vi "_emi_GFV Loop Running.vi"(0 "Loop Index/Numb":u16, 1 "Action(Get Index)":T1=enum."Get index", 7 "Loop Running In(F)":bool, 11 "error in (no error)":errorcluster) -> (4 "Index out":u16, 8 "Loop Running Out":bool, 10 "Size":i32, 15 "error out":errorcluster)   [LabVIEW 2011]
uses:
  _emi_Loop control int action.ctl
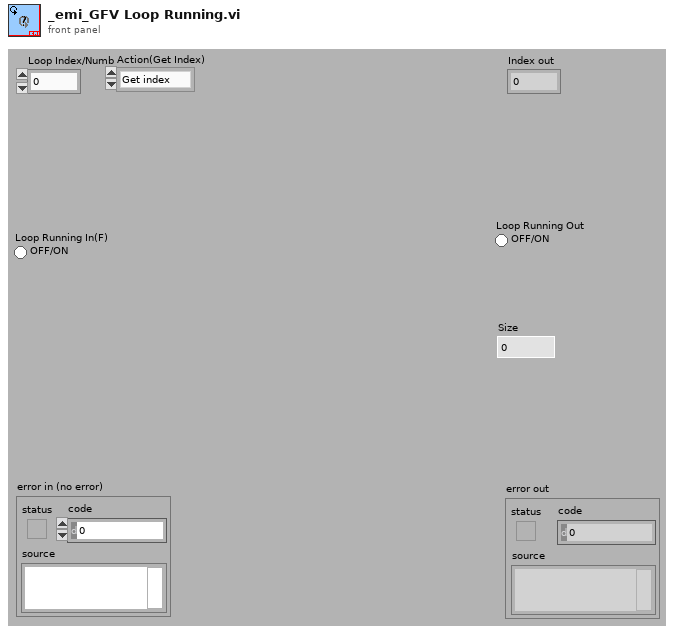
[diagram p1: front panel]
types:
  T1 = typedef "_emi_Loop control int action.ctl" = enum16{"Init index", "Get index", "Set index", "Get Size"}
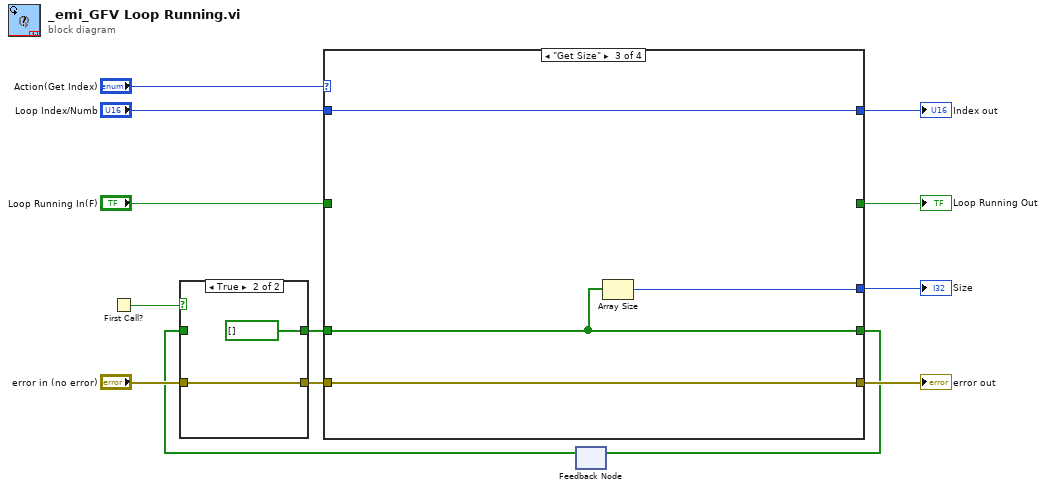
[diagram p0: block diagram]
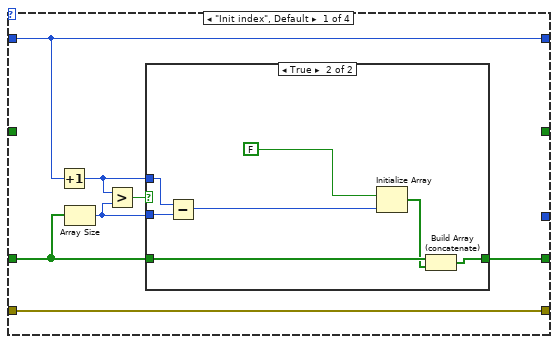
[diagram p2: hidden frame]
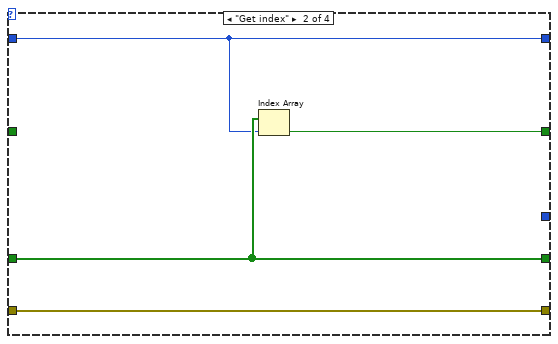
[diagram p4: hidden frame]
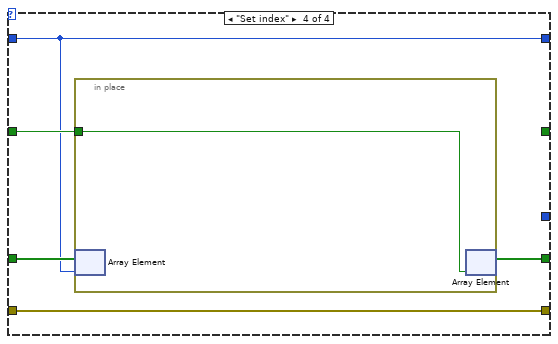
[diagram p5: hidden frame]
diagram:
  n1 = First Call?() -> (First Call?: T/F=w10:bool)
  n2 = feedback #1() -> (w4:bool[])  [unwired: 1 in]
  n3 = case shown="True" w10 {
    tunnel: [w15 w17] -> w12
    tunnel: "error in (no error)" -> [w15 w17]
    tunnel: [w14 bool[] []] -> w5
    tunnel: w4 -> [w14 _]
    frame False {
    }
    frame True {
    }
  }
  n4 = case shown="\"Get Size\"" "Action(Get Index)" {
    tunnel: [w24 w36 w40 w45] -> w13
    tunnel: w12 -> [w24 w36 w40 w45]
    tunnel: [w23 w34 w39 w41] -> w9
    tunnel: "Loop Index/Numb" -> [w23 w34 w39 w41]
    tunnel: [w19 w35 w38 w43] -> w6
    tunnel: w5 -> [w18 w35 w38 w44]
    tunnel: [_ w33 _ _] -> w3
    tunnel: "Loop Running In(F)" -> [_ _ _ w42]
    tunnel: [_ _ w37 _] -> w1
    frame "Init index", Default {
      n5 = Increment(x=w23) -> (x+1=w20:u16)
      n6 = Array Size(array=w18) -> (size(s)=w21:i32)
      n7 = Greater?(x=w20, y=w21) -> (0:w22:bool)
      n8 = case shown="True" w22 {
        tunnel: w21 -> [_ w31]
        tunnel: w20 -> [_ w32]
        tunnel: [w25 w26] -> w19
        tunnel: w18 -> [w25 w28]
        frame False {
        }
        frame True {
          n9 = Subtract(x=w32, y=w31) -> (x-y=w30:i32)
          n10 = Initialize Array(FALSE, w30) -> (w27:bool[])
          n11 = Build Array (concatenate)(w28, w27) -> (w26:bool[])
        }
      }
    }
    frame "Get index" {
      n12 = Index Array(array=w35, index=w34) -> (element=w33:bool)
    }
    frame "Get Size" {
      n13 = Array Size(array=w38) -> (size(s)=w37:i32)
    }
    frame "Set index" {
      n14 = in-place {
        in-place-border: w42 -> [w46]
        n15 = in-place-array #2(w44, w41) -> ()  [unwired: 1 out]
        n16 = in-place-array #2(w46) -> (w43:bool[])  [unwired: 1 out]
      }
    }
  }
  "error out" <- w13
  "Index out" <- w9
  "Loop Running Out" <- w3
  "Size" <- w1
  n17 = feedback-in #1(w6) -> ()
